vi "SubVI_SA_Init.vi"(8 "error in (no error)":errorcluster, 10 "CenterFreq(GHz) 2":dbl=28.0, 11 "VISA resource name":refnum<visa-resource-name>="TCPIP0::192.168.100.230::inst0::INSTR") -> (0 "error out 2":errorcluster, 3 "VISA resource name out":refnum<visa-resource-name>, 4 "Marker Response 2":dbl format="%.3f")   [LabVIEW 2023]
uses:
  CTL/Spectrum_type.ctl
  Anritsu Signal Analyzer Series/Public/Configure/Configure Frequency (Center Span).vi
  Anritsu Signal Analyzer Series/Public/Data/Read Marker (Active Marker).vi
  Anritsu Signal Analyzer Series/Anritsu Signal Analyzer Series.lvlib
panel:
  # "TCPIP::192.168.100.230::INSTR"
  # "TCPIP0::192.168.100.230::inst0::INSTR"
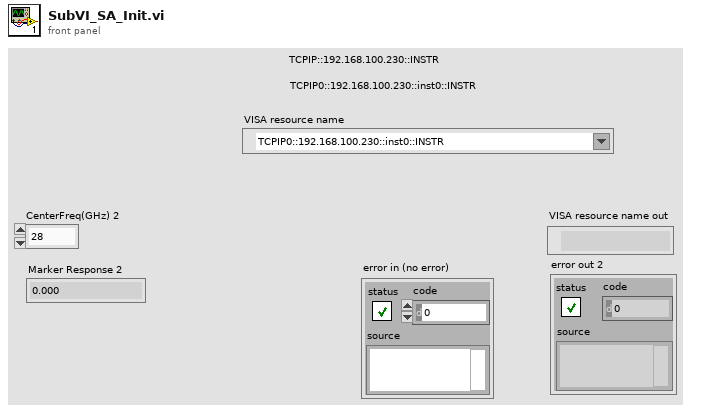
[diagram p1: front panel]
types:
  T1 = typedef "Spectrum_type.ctl" = enum16{"anritsu", "keysight"}
  T2 = cluster{"Width Frequency (1000000Hz)":dbl, "Width Point (100)":i32, "Width (0:0.5 div)":i32}
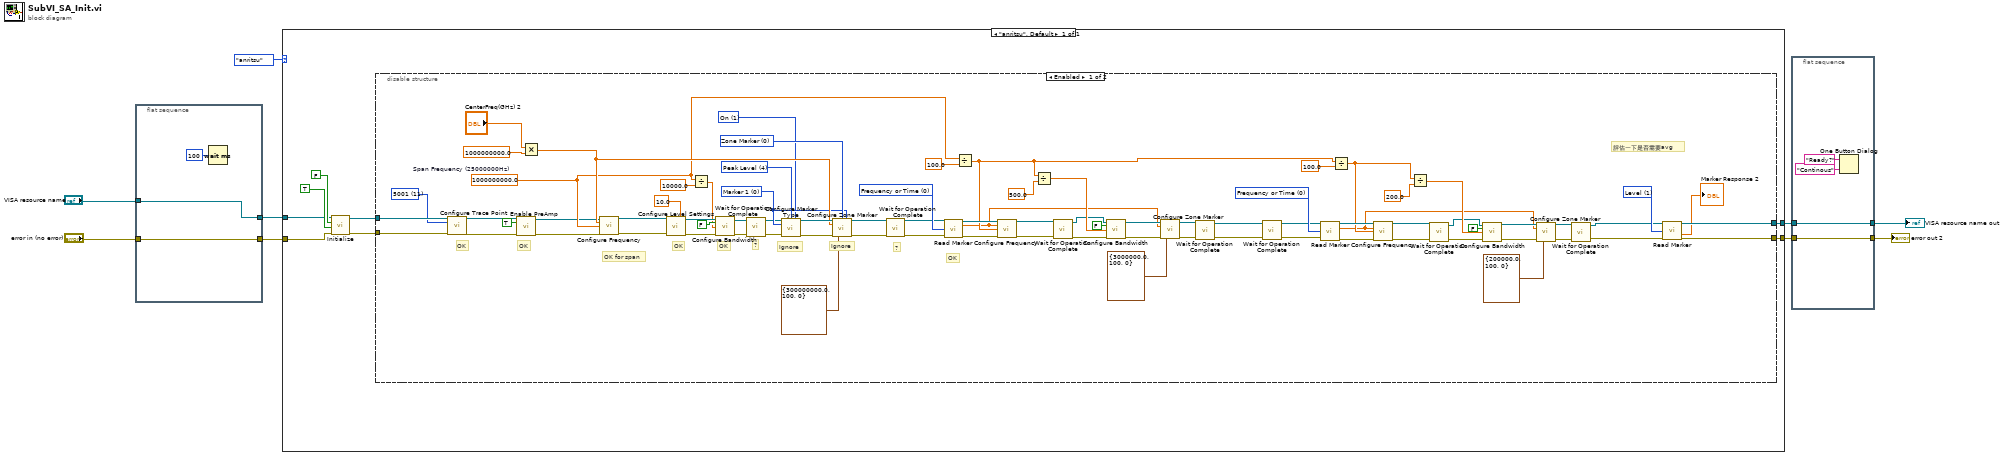
[diagram p0: block diagram]
diagram:
  n1 = flat-sequence {
    tunnel: "VISA resource name" -> [w12]
    tunnel: "error in (no error)" -> [w11]
    tunnel: [w12] -> w7
    tunnel: [w11] -> w6
    frame #0 {
      n2 = Wait (ms)(milliseconds to wait=u32 100) -> ()  [unwired: 1 out]
    }
  }
  n3 = case shown="\"anritsu\", Default" Spectrum_type."anritsu" {
    tunnel: w7 -> [w16]
    tunnel: w6 -> [w15]
    tunnel: [w14] -> w5
    tunnel: [w13] -> w4
    frame "anritsu", Default {
      n4 = call "Initialize.vi"("error in (no error)"=w15, "Reset (T:True)"=TRUE, "ID Query (T:True)"=FALSE, "VISA resource name"=w16) -> ("error out"=w19:errorcluster, "VISA resource name out"=w20:refnum<visa-resource-name>)  [unwired: 6 in]
      n5 = disable-structure shown="Enabled" {
        disable-tunnel: w20 -> [w84 w103]
        disable-tunnel: w19 -> [w83 w102]
        disable-tunnel: [w56 w103] -> w14
        disable-tunnel: [w55 w102] -> w13
        frame Enabled {
          w24 = 11 items=["11", "21", "41", "51", "101", "201", "251", "401", "501", "1001", "2001", "5001", "10001"] ("Trace Points (12:10001)")
          w25 = 1 items=["Off", "On"] ("Tracking (0:Off)")
          w54 = 0 items=["Frequency or Time", "Level", "Position"] ("Marker Type (0:Frequency or Time)")
          w81 = 0 items=["Frequency or Time", "Level", "Position"] ("Marker Type (0:Frequency or Time)")
          w85 = 1 items=["Frequency or Time", "Level", "Position"] ("Marker Type (0:Frequency or Time)")
          w88 = 0 items=["Zone Marker", "Spot Marker"] ("Marker Type (0:Zoom Marker)")
          w91 = 4 items=["Total", "Average", "Integral Power", "Power Density", "Peak Level"] ("Marker Type (2:Integral Power)")
          w86 = 0 items=["Marker 1", "Marker 2", "Marker 3", "Marker 4", "Marker 5", "Marker 6", "Marker 7", "Marker 8", "Marker 9", "Marker 10"] ("Marker Target (0:Marker 1)")
          w78 = 1000000000.0  # Span Frequency (25000000Hz)
          # "OK"
          # "?"
          # "Ignore"
          # "Ignore"
          # "?"
          # "OK"
          # "OK"
          # "OK for span"
          # "OK"
          # "OK"
          # "評估一下是否需要avg"
          n6 = call "Configure Trace Point.vi"("VISA resource name"=w84, "Trace Points (12:10001)"=w24, "error in (no error)"=w83) -> ("VISA resource name out"=w30:refnum<visa-resource-name>, "error out"=w27:errorcluster)  [unwired: 11 in]
          n7 = call "Enable PreAmp.vi"("VISA resource name"=w30, "Enable PreAmp (F:Disable)"=TRUE, "error in (no error)"=w27) -> ("VISA resource name out"=w29:refnum<visa-resource-name>, "error out"=w28:errorcluster)  [unwired: 11 in]
          n8 = Multiply(x="CenterFreq(GHz) 2", y=1000000000.0 ("Center Frequency (3000000000Hz)")) -> (x*y=w87:dbl)
          n9 = call-poly "Configure Frequency.vi"("VISA resource name"=w29, "Center Frequency (3000000000Hz)"=w87, "Span Frequency (25000000Hz)"=w78, "error in (no error)"=w28) -> ("VISA resource name out"=w99:refnum<visa-resource-name>, "error out"=w98:errorcluster)  [unwired: 10 in]
          n10 = call "Configure Level Settings.vi"("VISA resource name"=w99, "Reference Level (-10.00dBm)"=10.0, "error in (no error)"=w98) -> ("VISA resource name out"=w96:refnum<visa-resource-name>, "error out"=w95:errorcluster)  [unwired: 11 in]
          n11 = Divide(x=w78, y=10000.0) -> (x/y=w92:dbl)
          n12 = call "Configure Bandwidth.vi"("VISA resource name"=w96, "Auto Resolution Bandwidth  (T:Enable)"=FALSE, "Resolution Bandwidth (300:300Hz)"=w92, "error in (no error)"=w95) -> ("VISA resource name out"=w67:refnum<visa-resource-name>, "error out"=w70:errorcluster)  [unwired: 10 in]
          n13 = call "Wait for Operation Complete.vi"("error in (no error)"=w70, "VISA resource name"=w67) -> ("error out"=w69:errorcluster, "VISA resource name out"=w68:refnum<visa-resource-name>)  [unwired: 8 in]
          n14 = call "Configure Marker Type.vi"("VISA resource name"=w68, "Marker Type (2:Integral Power)"=w91, "Tracking (0:Off)"=w25, "Marker Target (0:Marker 1)"=w86, "error in (no error)"=w69) -> ("VISA resource name out"=w90:refnum<visa-resource-name>, "error out"=w89:errorcluster)  [unwired: 9 in]
          n15 = call "Configure Zone Marker.vi"("VISA resource name"=w90, "Marker Type (0:Zoom Marker)"=w88, "Marker (0:Marker 1)"=w86, "Zone Marker Frequency (3000000000Hz)"=w87, "error in (no error)"=w89, "Zone Width"=T2 {"Width Frequency (1000000Hz)"=300000000.0, "Width Point (100)"=100, "Width (0:0.5 div)"=0}) -> ("VISA resource name out"=w60:refnum<visa-resource-name>, "error out"=w59:errorcluster)  [unwired: 8 in]
          n16 = call "Wait for Operation Complete.vi"("error in (no error)"=w59, "VISA resource name"=w60) -> ("error out"=w58:errorcluster, "VISA resource name out"=w57:refnum<visa-resource-name>)  [unwired: 8 in]
          n17 = call-poly "Read Marker.vi"("VISA resource name"=w57, "Marker Type (0:Frequency or Time)"=w81, "error in (no error)"=w58) -> ("VISA resource name out"=w80:refnum<visa-resource-name>, "Marker_X Response"=w22:dbl, "error out"=w79:errorcluster)  [unwired: 9 in, 1 out]
          n18 = Divide(x=w78, y=100.0) -> (x/y=w31:dbl)
          n19 = call-poly "Configure Frequency.vi"("VISA resource name"=w80, "Center Frequency (3000000000Hz)"=w22, "Span Frequency (25000000Hz)"=w31, "error in (no error)"=w79) -> ("VISA resource name out"=w66:refnum<visa-resource-name>, "error out"=w65:errorcluster)  [unwired: 10 in]
          n20 = Divide(x=w31, y=500.0) -> (x/y=w75:dbl)
          n21 = call "Wait for Operation Complete.vi"("error in (no error)"=w65, "VISA resource name"=w66) -> ("error out"=w64:errorcluster, "VISA resource name out"=w63:refnum<visa-resource-name>)  [unwired: 8 in]
          n22 = call "Configure Bandwidth.vi"("VISA resource name"=w63, "Auto Resolution Bandwidth  (T:Enable)"=FALSE, "Resolution Bandwidth (300:300Hz)"=w75, "error in (no error)"=w64) -> ("VISA resource name out"=w73:refnum<visa-resource-name>, "error out"=w72:errorcluster)  [unwired: 10 in]
          n23 = call "Configure Zone Marker.vi"("VISA resource name"=w73, "Zone Marker Frequency (3000000000Hz)"=w22, "error in (no error)"=w72, "Zone Width"=T2 {"Width Frequency (1000000Hz)"=3000000.0, "Width Point (100)"=100, "Width (0:0.5 div)"=0}) -> ("VISA resource name out"=w61:refnum<visa-resource-name>, "error out"=w62:errorcluster)  [unwired: 10 in]
          n24 = call "Wait for Operation Complete.vi"("error in (no error)"=w62, "VISA resource name"=w61) -> ("error out"=w35:errorcluster, "VISA resource name out"=w34:refnum<visa-resource-name>)  [unwired: 8 in]
          n25 = call "Wait for Operation Complete.vi"("error in (no error)"=w35, "VISA resource name"=w34) -> ("error out"=w37:errorcluster, "VISA resource name out"=w36:refnum<visa-resource-name>)  [unwired: 8 in]
          n26 = call-poly "Read Marker.vi"("VISA resource name"=w36, "Marker Type (0:Frequency or Time)"=w54, "error in (no error)"=w37) -> ("VISA resource name out"=w53:refnum<visa-resource-name>, "Marker_X Response"=w21:dbl, "error out"=w52:errorcluster)  [unwired: 9 in, 1 out]
          n27 = Divide(x=w31, y=100.0) -> (x/y=w50:dbl)
          n28 = call-poly "Configure Frequency.vi"("VISA resource name"=w53, "Center Frequency (3000000000Hz)"=w21, "Span Frequency (25000000Hz)"=w50, "error in (no error)"=w52) -> ("VISA resource name out"=w43:refnum<visa-resource-name>, "error out"=w42:errorcluster)  [unwired: 10 in]
          n29 = Divide(x=w50, y=200.0) -> (x/y=w48:dbl)
          n30 = call "Wait for Operation Complete.vi"("error in (no error)"=w42, "VISA resource name"=w43) -> ("error out"=w41:errorcluster, "VISA resource name out"=w40:refnum<visa-resource-name>)  [unwired: 8 in]
          n31 = call "Configure Bandwidth.vi"("VISA resource name"=w40, "Auto Resolution Bandwidth  (T:Enable)"=FALSE, "Resolution Bandwidth (300:300Hz)"=w48, "error in (no error)"=w41) -> ("VISA resource name out"=w46:refnum<visa-resource-name>, "error out"=w45:errorcluster)  [unwired: 10 in]
          n32 = call "Configure Zone Marker.vi"("VISA resource name"=w46, "Zone Marker Frequency (3000000000Hz)"=w21, "error in (no error)"=w45, "Zone Width"=T2 {"Width Frequency (1000000Hz)"=200000.0, "Width Point (100)"=100, "Width (0:0.5 div)"=0}) -> ("VISA resource name out"=w38:refnum<visa-resource-name>, "error out"=w39:errorcluster)  [unwired: 10 in]
          n33 = call "Wait for Operation Complete.vi"("error in (no error)"=w39, "VISA resource name"=w38) -> ("error out"=w32:errorcluster, "VISA resource name out"=w33:refnum<visa-resource-name>)  [unwired: 8 in]
          n34 = call-poly "Read Marker.vi"("VISA resource name"=w33, "Marker Type (0:Frequency or Time)"=w85, "error in (no error)"=w32) -> ("VISA resource name out"=w56:refnum<visa-resource-name>, "Marker_Y Response 2"=→"Marker Response 2":dbl, "error out"=w55:errorcluster)  [unwired: 9 in, 1 out]
        }
        frame Disabled {
        }
      }
    }
  }
  n35 = flat-sequence {
    tunnel: w5 -> [w107]
    tunnel: w4 -> [w106]
    tunnel: [w107] -> w3
    tunnel: [w106] -> w2
    frame #0 {
      n36 = One Button Dialog(message="Ready?", button name ("OK")="Continous") -> ()  [unwired: 1 out]
    }
  }
  "VISA resource name out" <- w3
  "error out 2" <- w2
